vi "Set Channel Value (Alpha).vi"(8 "error in (no error)":errorcluster, 10 "Value":u8, 11 "ARGB Image in":T1) -> (0 "error out":errorcluster, 3 "ARGB Image":T1)   [LabVIEW 2020, in "image.lvlib"]
doc: "Set the channel of an ARGB image to a single value."
uses:
  image.lvlib
  ARGB Image.ctl
  ARGBChannels.ctl
  <vilib>/Utility/error.llb/Error Cluster From Error Code.vi
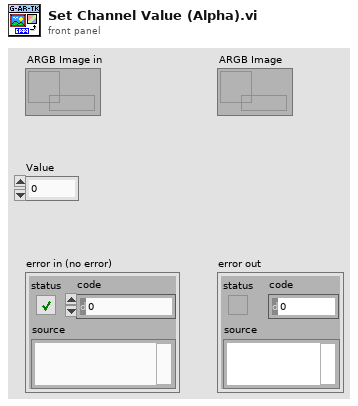
[diagram p1: front panel]
types:
  T1 = typedef "image.lvlib/ARGB Image.ctl" = refnum<data-value>
  T2 = typedef "image.lvlib/ARGBChannels.ctl" = enum8{"Blue", "Green", "Red", "Alpha"}
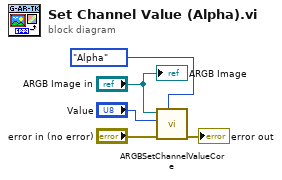
[diagram p0: block diagram]
diagram:
  n1 = call "ARGBSetChannelValueCore.vi"("Channel"=ARGBChannels."Alpha" ("Extract_Operation"), "error in (no error)"="error in (no error)", "Value"="Value", "Src in"="ARGB Image in") -> ("error out"=→"error out":errorcluster)  [unwired: 7 in]
  "ARGB Image" <- "ARGB Image in"
